vi "Pre Launch Init Correct.vi"(0 "Device in":refnum<class "Device.lvclass">, 5 "error in (no error)":errorcluster) -> (14 "Device out":refnum<class "Device.lvclass">, 19 "error out":errorcluster)   [LabVIEW 2014, in "DAQ Device.lvlib" / "Device.lvclass"]
uses:
  Device.lvclass
  DAQ Device/Cfg Msg.ctl
  <vilib>/ActorFramework/Actor/Actor.lvclass/Actor.ctl
  Device.lvclass/Device.ctl
  Devices/Configurable Device/Configurable Device.lvclass/Configurable Device.ctl
  Controller/Messages/Device Configuration/Get Serialized Device Configuration MSG.lvclass/Get Serialized Device Configuration MSG.ctl
  <vilib>/ActorFramework/Message Enqueuer/Message Enqueuer.lvclass/Message Enqueuer.ctl
  Messages/Generic CVT Init/Generic Init CVT Message.lvclass/Generic Init CVT Message.ctl
  Messages/Generic CVT Init/Write DevID.vi
  Messages/Generic CVT Init/Write SP.vi
  Devices/Configurable Device/Read ID.vi
  Devices/Configurable Device/Accessors/Read type.vi
  Devices/Configurable Device/Accessors/Read label.vi
  Devices/Configurable Device/Accessors/Read SN.vi
  Devices/Configurable Device/Read controller_.vi
  Devices/Configurable Device/Accessors/Read Addr.vi
  Devices/Configurable Device/Accessors/Read Model.vi
  Controller/Messages/Device Configuration/Write cfg cluster.vi
  Controller/xGlobal Data.vi
  <vilib>/ActorFramework/Message Priority Queue/Priority Enqueue.vi
  Devices/Configurable Device/Configurable Device.lvclass
  <vilib>/ActorFramework/Actor/Actor.lvclass
  <vilib>/ActorFramework/Message Enqueuer/Message Enqueuer.lvclass
  Controller/Messages/Device Configuration/Get Serialized Device Configuration MSG.lvclass
  Messages/Generic CVT Init/Generic Init CVT Message.lvclass
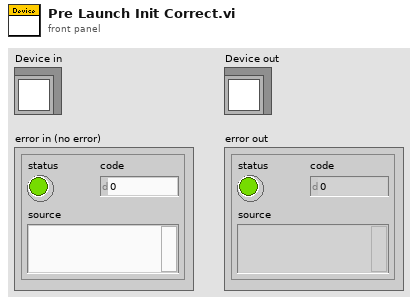
[diagram p1: front panel]
types:
  T1 = typedef "Cfg Msg.ctl" = cluster{"ID":string, "type":string, "label":string, "SN":string, "controller_":bool, "Addr":string, "Model":string}
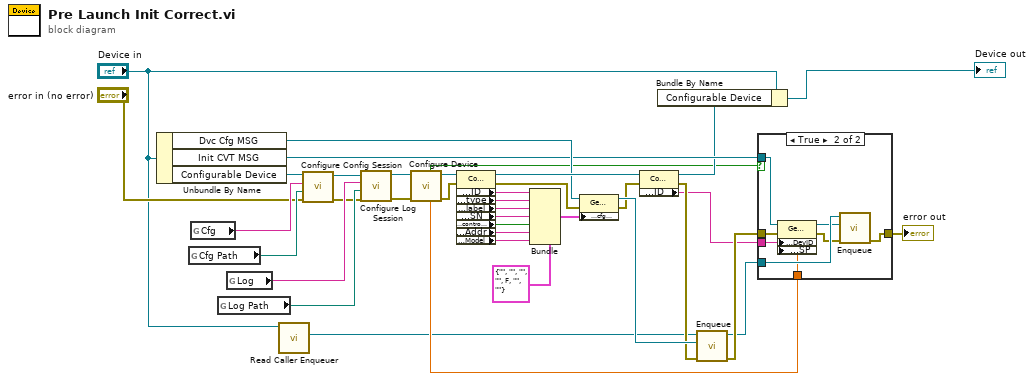
[diagram p0: block diagram]
diagram:
  n1 = Unbundle By Name("Device in") -> ("Dvc Cfg MSG"=w31:refnum<class "Get Serialized Device Configuration MSG.lvclass">, "Init CVT MSG"=w8:refnum<class "Generic Init CVT Message.lvclass">, "Configurable Device"=w17:refnum<class "Configurable Device.lvclass">)
  n2 = global read "xGlobal Data.vi" "Cfg Path"() -> (w22:path)
  n3 = global read "xGlobal Data.vi" "Cfg"() -> (w21:string)
  n4 = global read "xGlobal Data.vi" "Log Path"() -> (w19:path)
  n5 = global read "xGlobal Data.vi" "Log"() -> (w20:string)
  n6 = call <vilib>:"Read Caller Enqueuer.vi"("Actor"="Device in") -> ("Caller Enqueuer"=w2:refnum<class "Message Enqueuer.lvclass">)  [unwired: 10 in]
  n7 = call "Configure Config Session.vi"("error in (no error)"="error in (no error)", "Path"=w22, "Ref Name"=w21, "Configurable Device in"=w17) -> ("error out"=w16:errorcluster, "Configurable Device out"=w15:refnum<class "Configurable Device.lvclass">)  [unwired: 6 in]
  n8 = call "Configure Log Session.vi"("error in (no error)"=w16, "Path"=w19, "Ref Name"=w20, "Configurable Device in"=w15) -> ("error out"=w14:errorcluster, "Configurable Device out"=w13:refnum<class "Configurable Device.lvclass">)  [unwired: 6 in]
  n9 = call-dynamic "Configure Device.vi"("error in"=w14, "Device in"=w13) -> ("error out"=w37:errorcluster, "Device out"=w23:refnum<class "Configurable Device.lvclass">, "SP"=w7:dbl, "Settable?"=w3:bool)  [unwired: 6 in]
  n10 = property class="Configurable Device"(reference=w23, error in=w37) -> (reference out=w35:refnum<class "Configurable Device.lvclass">, error out=w38:errorcluster, "Accessors:ID"=w24:string, "Accessors:type"=w25:string, "Accessors:label"=w26:string, "Accessors:SN"=w27:string, "Accessors:controller_"=w28:bool, "Accessors:Addr"=w29:string, "Accessors:Model"=w36:string)
  n11 = Bundle(cluster=T1 {"ID"="", "type"="", "label"="", "SN"="", "controller_"=FALSE, "Addr"="", "Model"=""}, "ID"=w24, "type"=w25, "label"=w26, "SN"=w27, "controller_"=w28, "Addr"=w29, "Model"=w36) -> (w32:T1)
  n12 = property class="Get Serialized Device Configura"(reference=w31, error in=w38, "Accessors:cfg cluster"=w32) -> (reference out=w34:refnum<class "Get Serialized Device Configuration MSG.lvclass">, error out=w33:errorcluster)
  n13 = property class="Configurable Device"(reference=w35, error in=w33) -> (reference out=w5:refnum<class "Configurable Device.lvclass">, error out=w9:errorcluster, "Accessors:ID"=w6:string)
  n14 = Bundle By Name(cluster="Device in", "Configurable Device"=w5) -> (→"Device out":refnum<class "Device.lvclass">)
  n15 = call <vilib>:"Enqueue.vi"("error in (no error)"=w9, "Message"=w34, "Message Enqueuer in"=w2) -> ("error out"=w10:errorcluster, "Message Enqueuer out"=w4:refnum<class "Message Enqueuer.lvclass">)  [unwired: 7 in]
  n16 = case shown="True" w3 {
    tunnel: w4 -> [_ w47]
    tunnel: w8 -> [_ w46]
    tunnel: w6 -> [_ w45]
    tunnel: w7 -> [_ w44]
    tunnel: w10 -> [w39 w41]
    tunnel: [w39 w40] -> w11
    frame False {
    }
    frame True {
      n17 = property class="Generic Init CVT Message"(reference=w46, error in=w41, "Accessors:DevID"=w45, "Accessors:SP"=w44) -> (reference out=w43:refnum<class "Generic Init CVT Message.lvclass">, error out=w42:errorcluster)
      n18 = call <vilib>:"Enqueue.vi"("error in (no error)"=w42, "Message"=w43, "Message Enqueuer in"=w47) -> ("error out"=w40:errorcluster)  [unwired: 7 in, 1 out]
    }
  }
  "error out" <- w11
